vi "turn_upto_45.vi"   [LabVIEW 2014, in "mit2.lvrbt"]
uses:
  mit2.lvrbt
  <vilib>/NXT/Hardware/Plugins/Tetrix DC Motor/TetrixDCMotorAddress.ctl
  <vilib>/NXT/NXTIO Xnodes/NXTIONodeSubVIs/TETRIX IO Move DC Motors.vi
  <vilib>/NXT/Dual Mode Library/Sensors/EV3_Gyro_Angle.vi
  <vilib>/NXT/NXTIO Xnodes/NXTIONodeSubVIs/TETRIX IO Stop DC Motors.vi
  <vilib>/NXT/NXTIO Xnodes/AddressXNode/NXTIOAddress.xnode
  <vilib>/NXT/Subs/LVHSConnector.ctl
  <vilib>/NXT/NXTIO Xnodes/NXTIOXNode/NXTIO.xnode
  <vilib>/NXT/LegoClasses/BrickReference/BrickReference.lvclass
types:
  T1 = typedef "TetrixDCMotorAddress.ctl" = i32
  T2 = cluster{"TetrixDCMotor":T1, "TetrixDCMotor 2":T1}
  T3 = typedef "LVHSConnector.ctl" = refnum<class "BrickReference.lvclass">
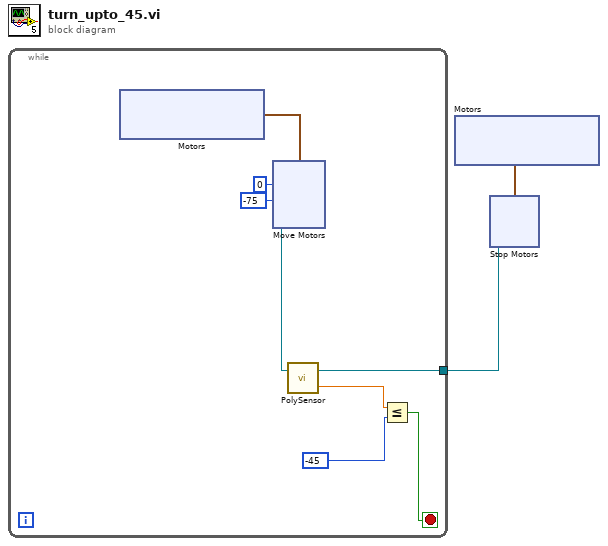
[diagram p0: block diagram]
diagram:
  n1 = while {
    tunnel: [w7] -> w1
    stop <- w3 stop-if-true
    n2 = xnode "Motors"() -> ("Motor"=w10:cluster{"TetrixDCMotor":T1, "TetrixDCMotor":T1})
    n3 = xnode "Move Motors"("Power/Speed 2"=i8 -75, "Power/Speed 1"=i8 0, "Motors"=w10) -> ("NXT/EV3"=w8:T3)  [unwired: 1 in]
    n4 = call-poly <vilib>:"PolySensor.vi"("NXT/EV3"=w8) -> ("Degrees"=w4:sgl, "NXT/EV3"=w7:T3)  [unwired: 2 in]
    n5 = Less Or Equal?(x=w4, y=-45) -> (x <= y?=w3:bool)
  }
  n6 = xnode "Motors"() -> ("Motor"=w2:cluster{"TetrixDCMotor":T1, "TetrixDCMotor":T1})
  n7 = xnode "Stop Motors"("Motors"=w2, "NXT/EV3"=w1) -> ()  [unwired: 1 out]
